vi "itemsym to string.vi"(11 "Item sym":i32[](array[numeric])=[37, 37, 38, 38]) -> (3 "Item sym string":string[](array[string]))   [LabVIEW 2012]
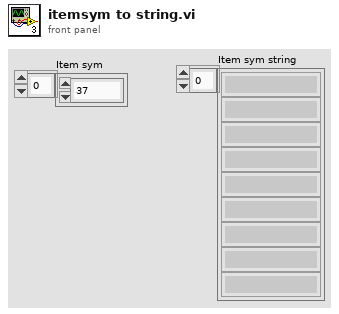
[diagram p1: front panel]
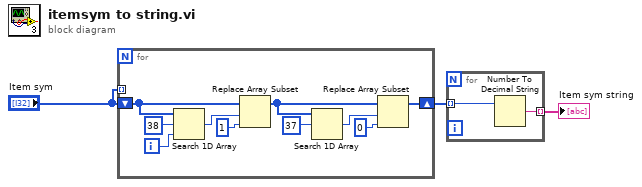
[diagram p0: block diagram]
diagram:
  n1 = for {
    tunnel: "Item sym" -> [_] mode=indexing
    shift-right: [w5] -> w2
    shift-left: "Item sym" -> [w6]
    i -> [w11]
    n2 = Search 1D Array(1D array=w6, element=38, start index (0)=w11) -> (index of element=w10:i32)
    n3 = Replace Array Subset(array=w6, new element=1 ("new element/subarray"), index=w10) -> (w4:i32[])
    n4 = Search 1D Array(1D array=w4, element=37) -> (index of element=w7:i32)  [unwired: 1 in]
    n5 = Replace Array Subset(array=w4, new element=0 ("new element/subarray"), index=w7) -> (w5:i32[])
  }
  n6 = for {
    tunnel: w2 -> [w15] mode=indexing
    tunnel: [w14] -> w1 mode=indexing
    n7 = Number To Decimal String(number=w15) -> (decimal integer string=w14:string)  [unwired: 1 in]
  }
  "Item sym string" <- w1
